vi "subDAQ_GetAI.vi"(8 "error in (no error)":errorcluster, 11 "AI line":tag="Dev1/ai0") -> (0 "error out":errorcluster, 3 "AI signal (V)":dbl format="%0.2f")   [LabVIEW 2015]
uses:
  <vilib>/DAQmx/read.llb/DAQmx Read (Analog DBL 1Chan 1Samp).vi
  <vilib>/DAQmx/create/channels.llb/DAQmx Create Channel (AI-Voltage-Basic).vi
  <vilib>/DAQmx/miscellaneous.llb/DAQmx Fill In Error Info.vi
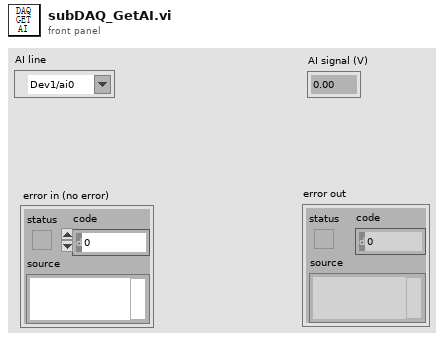
[diagram p1: front panel]
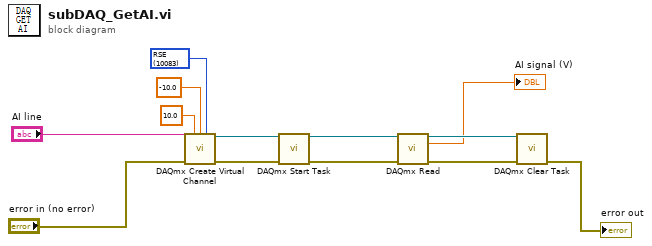
[diagram p0: block diagram]
diagram:
  w1 = 10083 items=["Default"=-1, "RSE"=10083, "NRSE"=10078, "Differential"=10106, "Pseudodifferential"=12529] ("input terminal configuration")
  n1 = call-poly <vilib>:"DAQmx Create Virtual Channel.vi"("maximum value"=10.0, "minimum value"=-10.0, "input terminal configuration"=w1, "physical channels"="AI line", "error in"="error in (no error)") -> ("task out"=w8:refnum<k21>, "error out"=w7:errorcluster)  [unwired: 4 in, 5 out]
  n2 = call <vilib>:"DAQmx Start Task.vi"("task/channels in"=w8, "error in"=w7) -> ("task out"=w9:refnum<k21>, "error out"=w10:errorcluster)  [unwired: 12 out]
  n3 = call-poly <vilib>:"DAQmx Read.vi"("task/channels in"=w9, "error in"=w10) -> ("task out"=w3:refnum<k21>, "data"=→"AI signal (V)":dbl, "error out"=w4:errorcluster)  [unwired: 11 in]
  n4 = call <vilib>:"DAQmx Clear Task.vi"("task in"=w3, "error in"=w4) -> ("error out"=→"error out":errorcluster)  [unwired: 13 out]
